vi "AMP_LMT_CHK.vi"(1 "Amplitude":dbl, 5 "error in":errorcluster) -> (14 "error out":errorcluster, 15 "Amplitude":dbl)   [LabVIEW 2018, in "PNA-X.lvlib"]
uses:
  PNA-X.lvlib
panel:
  in  "Limits":cluster{"AmpMax":dbl, "AmpMin":dbl}
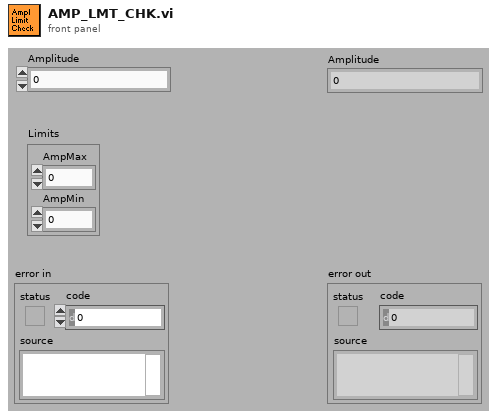
[diagram p1: front panel]
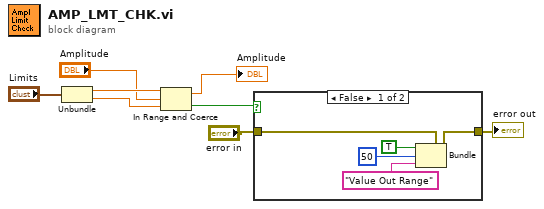
[diagram p0: block diagram]
diagram:
  n1 = Unbundle("Limits") -> ("AmpMax"=w7:dbl, "AmpMin"=w6:dbl)
  n2 = In Range and Coerce(upper limit=w7, x="Amplitude", lower limit=w6) -> (coerced(x)=→"Amplitude":dbl, In Range?=w2:bool)
  n3 = case shown="False" w2 {
    tunnel: "error in" -> [w12 w14]
    tunnel: [w13 w14] -> w3
    frame False {
      n4 = Bundle(cluster=w12, "status"=TRUE, "code"=50, "source"="Value Out Range") -> (w13:errorcluster)
    }
    frame True {
    }
  }
  "error out" <- w3
